vi "Heater_D2XX_2.vi"(8 "error in (no error) 2":errorcluster, 11 "Numeric 2":i32) -> (0 "error out 2":errorcluster)   [LabVIEW 2019]
uses:
  D2XX_HeaterStage/D2XX_HeaterStage.lvlib
  <userlib>/LevyLab/Relay Box/D2XX_Functions/D2XX_Functions.lvlib
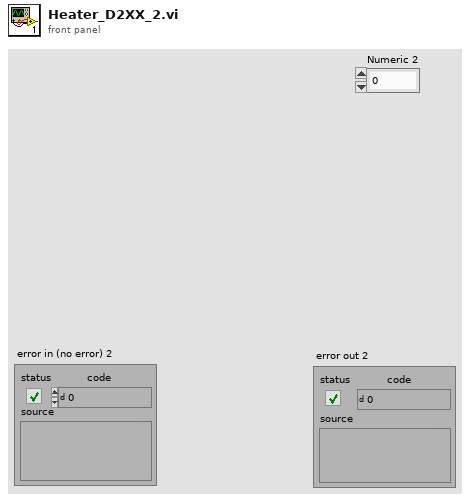
[diagram p1: front panel]
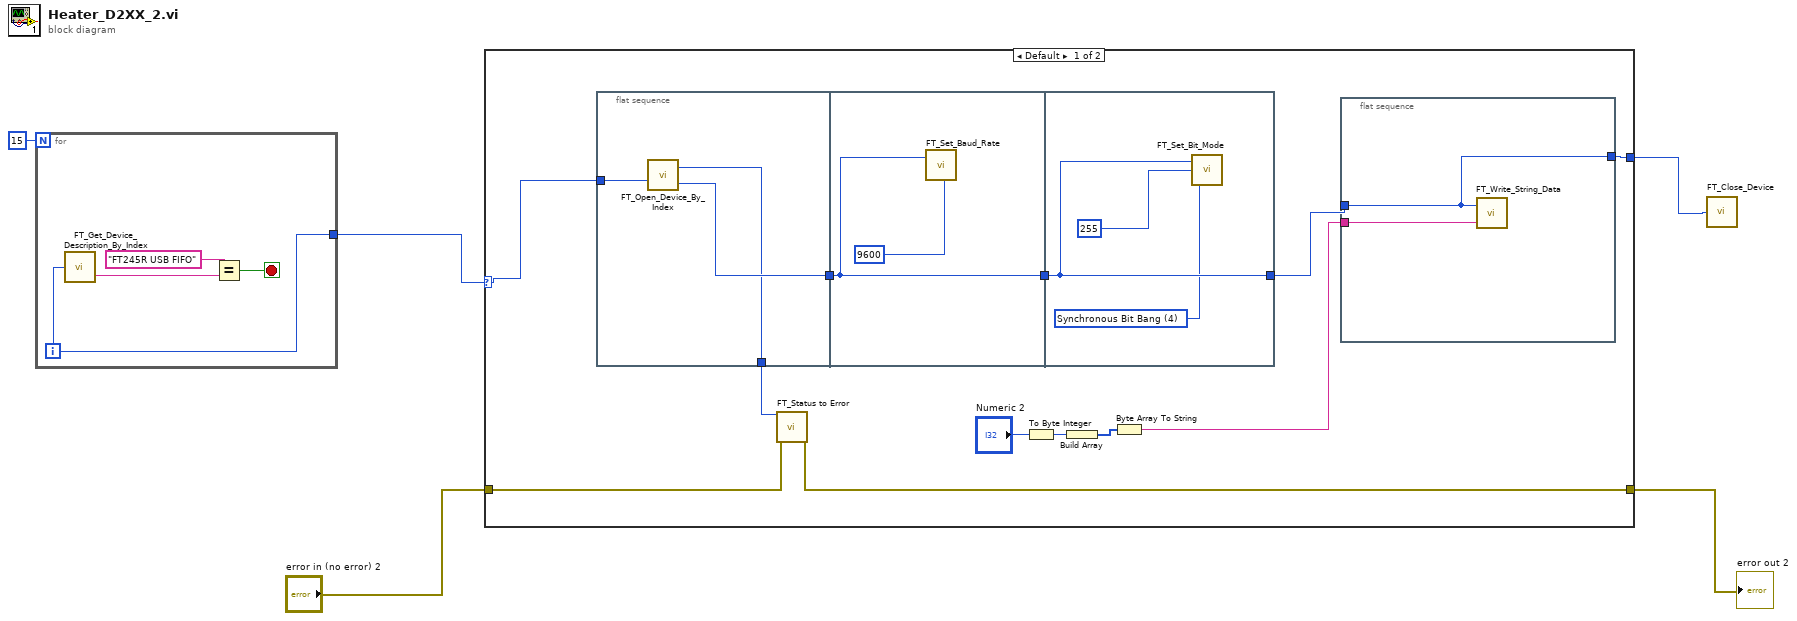
[diagram p0: block diagram]
diagram:
  n1 = for {
    N: 15 -> [_]
    tunnel: [w6] -> w2
    i -> [w6]
    stop <- w7 stop-if-true
    n2 = call "FT_Get_Device_Description_By_Index.vi"("Device Index"=w6) -> ("Device Description"=w8:string)  [unwired: 1 out]
    n3 = Equal?(x="FT245R USB FIFO", y=w8) -> (x = y?=w7:bool)
  }
  n4 = case shown="Default" w2 {
    selector: w2 -> [w16 w32]
    tunnel: [w11 w33] -> w3
    tunnel: "error in (no error) 2" -> [w12 w33]
    tunnel: [w15 w32] -> w1
    frame Default {
      n5 = flat-sequence {
        tunnel: w16 -> [w23]
        tunnel: [w24] -> w14
        tunnel: [w22] -> w10
        tunnel: w14 -> [w26]
        tunnel: [w26] -> w13
        tunnel: [w29] -> w18
        tunnel: w13 -> [w29]
        frame #0 {
          n6 = call "FT_Open_Device_By_Index.vi"("Device Index"=w23) -> ("FT_Status"=w22:u32, "Handle"=w24:u32)
        }
        frame #1 {
          n7 = call <userlib>:"FT_Set_Baud_Rate.vi"("Baud Rate"=u32 9600, "Handle"=w26) -> ()  [unwired: 1 out]
        }
        frame #2 {
          w27 = u8 4 items=["Reset Bit Mode"=0, "Asynchronous Bit Bang"=1, "MPSSE"=2, "Synchronous Bit Bang"=4, "MCU Host Bus Emulation"=8, "Fast Opto-Isolated Serial"=16, "CBUS Bit Bang"=32, "Single Channel 245 Synchronous FIFO"=64] ("Bit Mode")
          n8 = call <userlib>:"FT_Set_Bit_Mode.vi"("Bit Mode"=w27, "Bit Mode Mask"=u8 255, "Handle"=w29) -> ()  [unwired: 1 out]
        }
      }
      n9 = call "FT_Status to Error.vi"("error in (no error)"=w12, "Numeric"=w10) -> ("error out"=w11:errorcluster)  [unwired: 9 in]
      n10 = To Byte Integer(number="Numeric 2") -> (8bit integer=w21:i8)
      n11 = Build Array(w21) -> (w20:i8[])
      n12 = Byte Array To String(unsigned byte array=w20) -> (string=w19:string)
      n13 = flat-sequence {
        tunnel: w18 -> [w31]
        tunnel: [w31] -> w15
        tunnel: w19 -> [w30]
        frame #0 {
          n14 = call "FT_Write_String_Data.vi"("Buffer"=w30, "Handle"=w31) -> ()  [unwired: 2 out]
        }
      }
    }
    frame 1 {
    }
  }
  "error out 2" <- w3
  n15 = call "FT_Close_Device.vi"("Handle"=w1) -> ()  [unwired: 1 out]
